vi "CompressAndUpdate(Numeric).vi"(7 "force CVT update (false)":bool, 8 "error in":errorcluster, 9 "precision (6)":i16=6, 10 "Numeric":dbl, 11 "command or variable name":string) -> (0 "error out":errorcluster)   [LabVIEW 2011]
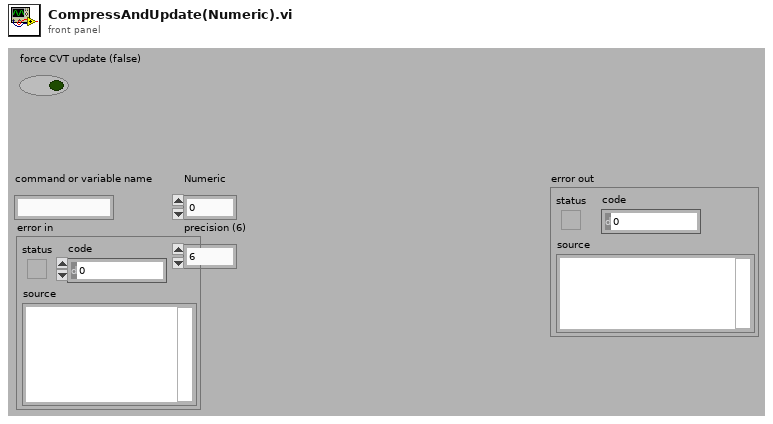
[diagram p1: front panel]
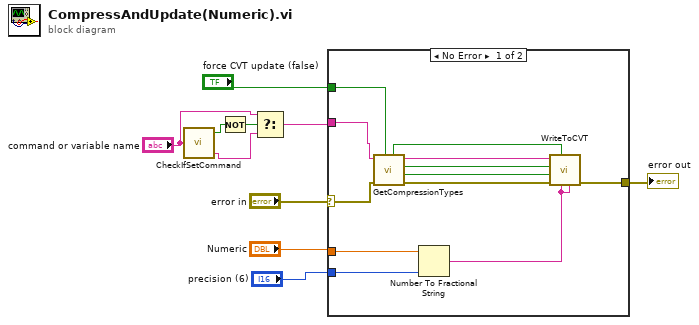
[diagram p0: block diagram]
diagram:
  n1 = call "CheckIfSetCommand.vi"("Command"="command or variable name") -> ("setCommand?"=w6:bool, "variable"=w3:string)  [unwired: 1 out]
  n2 = Not(x=w6) -> (.not. x?=w5:bool)
  n3 = Select(t="command or variable name", s=w5, f=w3) -> (s? t:f=w2:string)
  n4 = case shown="No Error" "error in" {
    selector: "error in" -> [w20 w23]
    tunnel: "Numeric" -> [w22 _]
    tunnel: "precision (6)" -> [w21 _]
    tunnel: w2 -> [w16 _]
    tunnel: [w11 w23] -> w7
    tunnel: "force CVT update (false)" -> [w13 _]
    frame No Error {
      n5 = call "GetCompressionTypes.vi"("force CVT update"=w13, "error in"=w20, "variable"=w16) -> ("error out"=w19:errorcluster, "non compressed"=w18:bool, "compressed"=w17:bool, "variable out"=w15:string, "force CVT update out"=w14:bool)  [unwired: 4 in]
      n6 = Number To Fractional String(number=w22, precision (6)=w21) -> (F-format string=w12:string)  [unwired: 2 in]
      n7 = call "WriteToCVT.vi"("non compressed string"=w12, "compressed string"=w12, "force CVT update"=w14, "error in"=w19, "non compressed"=w18, "compressed"=w17, "variable"=w15) -> ("error out"=w11:errorcluster)  [unwired: 4 in]
    }
    frame Error {
    }
  }
  "error out" <- w7
